vi "GetActiveChannelStatus.vi"(8 "error in":errorcluster, 11 "VISA resource name":refnum<visa-resource-name>) -> (0 "error out":errorcluster, 1 "Active channel status":i32, 2 "Active channel status string":string, 3 "VISA resource name out":refnum<visa-resource-name>)   [LabVIEW 2023, in "Thermotron 8800.lvlib"]
doc: "DCHN\nCommand name: Send active channel status\nCommand type: System status\nDescription: This command returns a byte value that describes which channels (1 through 4) are\nactive. The byte value ranges from 0 to 15 based on which channels are active. The\nbyte is defined below:\nBits 0 through 3\n1 Channel 1\n2 Channel 2\n4 Channel 3\n8 Channel 4\nSyntax: DCHN?\nData type: Coded byte\nQuery example 1: DCHN?\n8800 response: 5 (4 + 1 = channels 1 and 3 are active.)\nQuery example 2: DCHN?\n8800 response: 0 (No channels are active.)"
uses:
  Thermotron 8800.lvlib
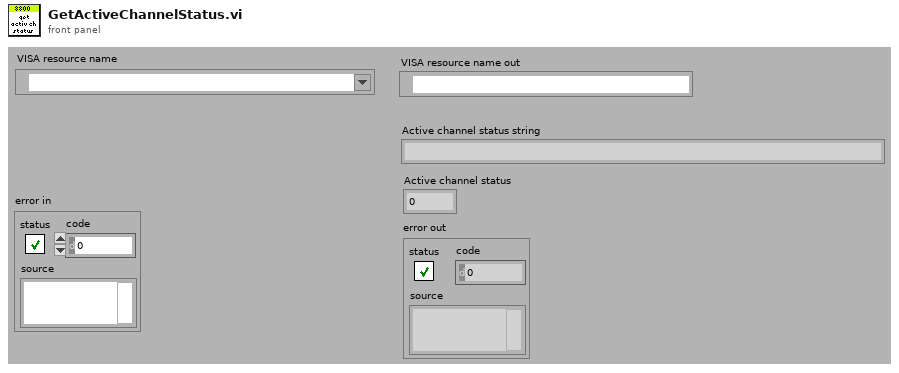
[diagram p1: front panel]
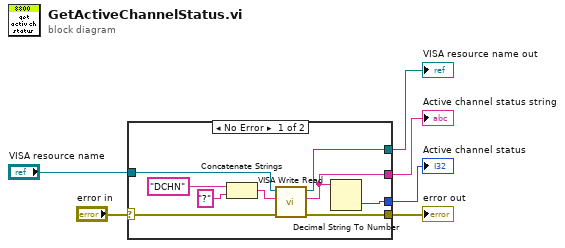
[diagram p0: block diagram]
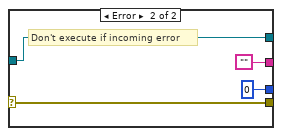
[diagram p2: hidden frame]
diagram:
  n1 = case shown="No Error" "error in" {
    selector: "error in" -> [w12 w19]
    tunnel: [w11 w19] -> w5
    tunnel: "VISA resource name" -> [w10 w18]
    tunnel: [w9 w18] -> w3
    tunnel: [w8 ""] -> w2
    tunnel: [w7 0] -> w1
    frame No Error {
      n2 = Concatenate Strings("DCHN" ("8800 Command"), "?" ("8800 Command")) -> (w13:string)
      n3 = call "VISA Write Read.vi"("error in (no error)"=w12, "8800 Command"=w13, "VISA Refnum in"=w10) -> ("error out"=w11:errorcluster, "read buffer"=w8:string, "VISA Refnum out"=w9:refnum<visa-resource-name>)  [unwired: 6 in]
      n4 = Decimal String To Number(string=w8) -> (number=w7:i32)  [unwired: 2 in, 1 out]
    }
    frame Error {
      # "Don't execute if incoming error"
    }
  }
  "error out" <- w5
  "VISA resource name out" <- w3
  "Active channel status string" <- w2
  "Active channel status" <- w1
